vi "Strip FileName.vi"(8 "error in":errorcluster, 10 "File Type":string, 11 "Filename":string) -> (0 "error out":errorcluster, 2 "Time Stamp":timestamp format="%<%Y/%m/%d>T", 3 "Distance (DBL)":dbl)   [LabVIEW 2024]
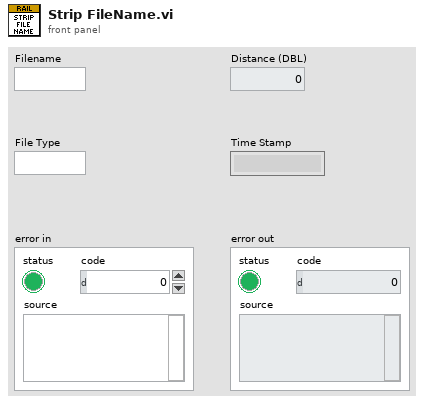
[diagram p1: front panel]
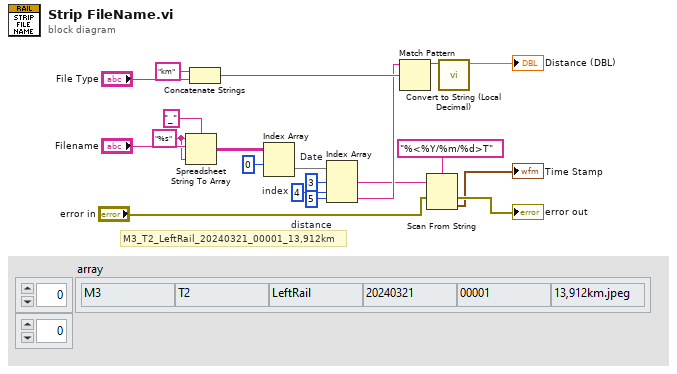
[diagram p0: block diagram]
diagram:
  w7 = 5  # distance
  w8 = 4  # index
  w9 = 3  # Date
  w13 = "%s" ("format string")
  # "M3_T2_LeftRail_20240321_00001_13,912km"
  n1 = Spreadsheet String To Array(delimiter (Tab)="_", format string=w13, spreadsheet string="Filename", array type (2D Dbl)=w13) -> (array=w12:string[][])
  n2 = Concatenate Strings("km" ("string"), "File Type") -> (w18:string)
  n3 = Index Array(array=w12, index (row)=0) -> (element=w10:string[])  [unwired: 1 in]
  n4 = Index Array(array=w10, index #1=w9, index #2=w8, index #3=w7) -> (element #1=w5:string, element #3=w6:string)  [unwired: 1 out]
  n5 = Match Pattern(string=w6, regular expression=w18) -> (before substring=w16:string)  [unwired: 1 in, 3 out]
  n6 = Scan From String(format string="%<%Y/%m/%d>T", input string=w5, error in="error in") -> (error out=→"error out":errorcluster, output 1=→"Time Stamp":timestamp)  [unwired: 2 in, 2 out]
  n7 = call "Convert to String (Local Decimal).vi"("Distance (String)"=w16) -> ("Distance (DBL)"=→"Distance (DBL)":dbl)  [unwired: 10 in]
